vi "Start SinglePlotPanel.vi"(8 "error in (no error)":errorcluster, 11 "SinglePlotPanel (type)":refnum<class "SinglePlotPanel.lvclass">) -> (0 "error out":errorcluster, 3 "SinglePlotPanel (running type)":refnum<class "SinglePlotPanel.lvclass">)   [LabVIEW 2021, in "MultiBluePlot.lvlib" / "SinglePlotPanel.lvclass"]
uses:
  SinglePlotPanel.lvclass
  SinglePlotPanel.lvclass/SinglePlotPanel.ctl
  <userlib>/Blue Origin/BluePlot (Open Source)/Classes/BluePlotHandle/BluePlotHandle.lvclass
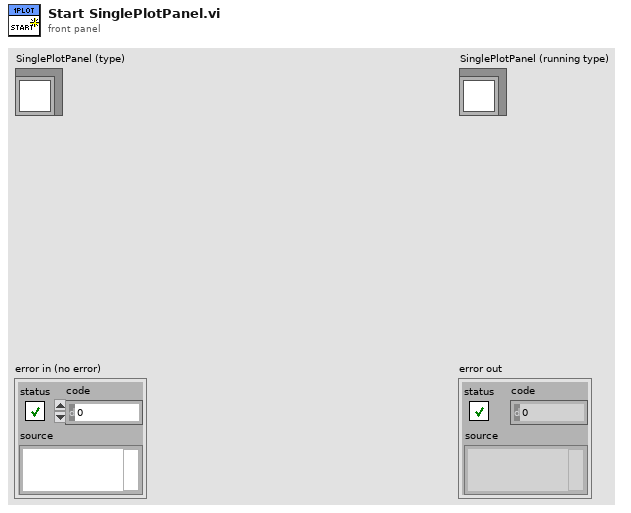
[diagram p1: front panel]
types:
  T1 = typedef "BluePlot.lvlib/BluePlotHandle.lvclass/Init Options.ctl" = cluster{"UI visible?":bool, "Update rate (ms)":u32, "visible sidebar?":bool, "time to plot (init)":dbl, "time to plot (max)":dbl, "config file start path":path}
  T2 = typedef "BluePlot.lvlib/BlueMultiPlot Inputs.ctl" = cluster{"plot menu":string[], "UE: ItemTag":refnum<user-event>}
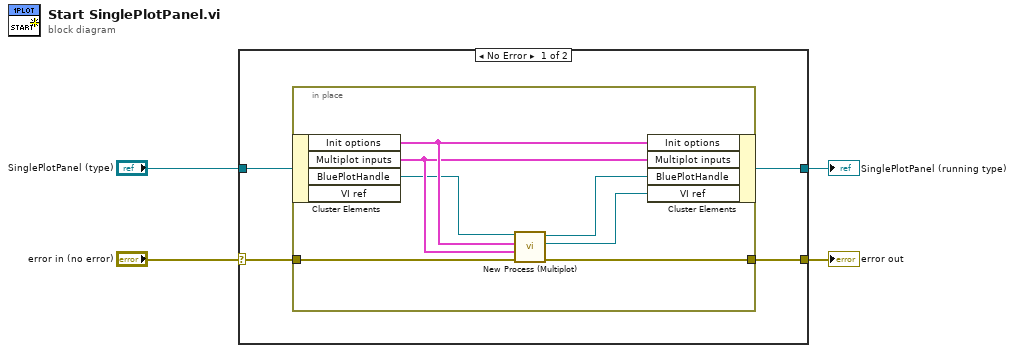
[diagram p0: block diagram]
diagram:
  n1 = case shown="No Error" "error in (no error)" {
    selector: "error in (no error)" -> [w7 w17]
    tunnel: [w6 w17] -> w3
    tunnel: [w5 w16] -> w1
    tunnel: "SinglePlotPanel (type)" -> [w8 w16]
    frame No Error {
      n2 = in-place {
        in-place-border: w7 -> [w13]
        in-place-border: [w12] -> w6
        n3 = in-place-cluster #1(w8) -> ("Init options"=w15:T1, "Multiplot inputs"=w14:T2, "BluePlotHandle"=w10:refnum<class "BluePlotHandle.lvclass">)  [unwired: 1 out]
        n4 = call <userlib>:"New Process (Multiplot).vi"("error in (no error)"=w13, "Multiplot inputs"=w14, "Init options"=w15, "BluePlotHandle in"=w10) -> ("error out"=w12:errorcluster, "VI ref"=w9:refnum<vi>, "BluePlotHandle out"=w11:refnum<class "BluePlotHandle.lvclass">)  [unwired: 5 in]
        n5 = in-place-cluster #1("Init options"=w15, "Multiplot inputs"=w14, "BluePlotHandle"=w11, "VI ref"=w9) -> (w5:refnum<class "SinglePlotPanel.lvclass">)
      }
    }
    frame Error {
    }
  }
  "error out" <- w3
  "SinglePlotPanel (running type)" <- w1
